vi "Write to Cell - Variant.vi"(8 "Column":i32=-1, 9 "Row":i32=-1, 10 "Value":variant, 11 "Excel Sheet in":refnum<class "Excel Sheet.lvclass">) -> (3 "Excel Sheet out":refnum<class "Excel Sheet.lvclass">)   [LabVIEW 2016, in "Excel Sheet.lvclass"]
uses:
  Excel Sheet.lvclass
  Excel Sheet.lvclass/Excel Sheet.ctl
panel:
  out "error out":errorcluster
  in  "error in (no error)":errorcluster
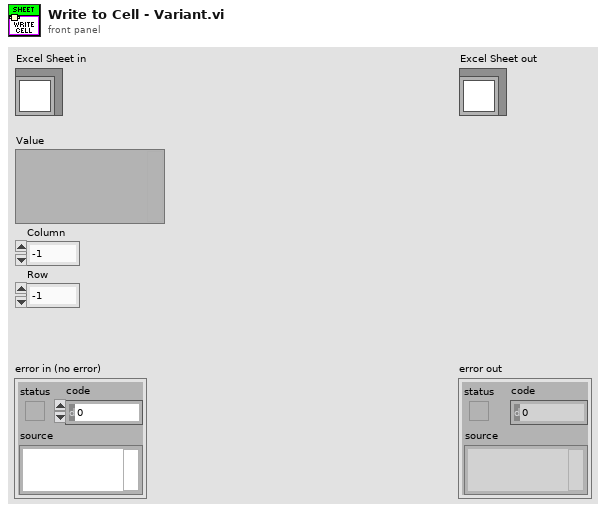
[diagram p1: front panel]
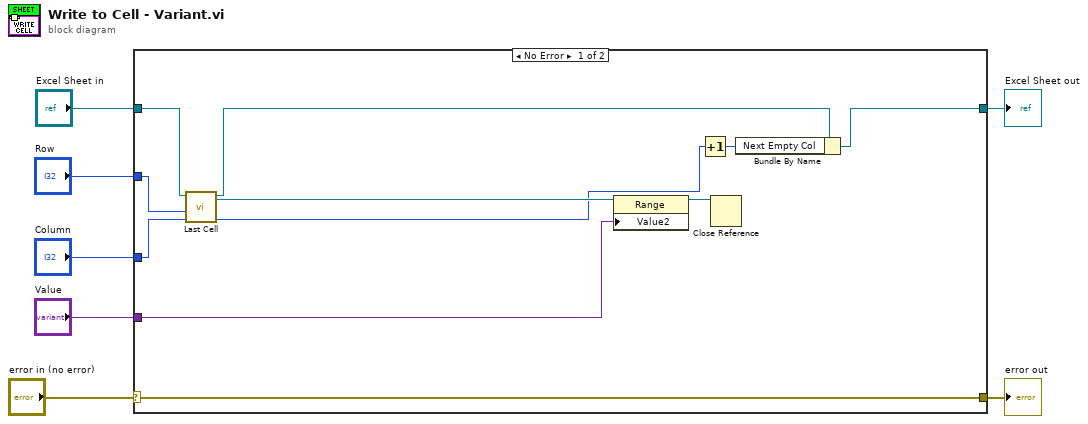
[diagram p0: block diagram]
diagram:
  n1 = case shown="No Error" "error in (no error)" {
    selector: "error in (no error)" -> [w18 w20]
    tunnel: [w18 w20] -> w6
    tunnel: [w16 w19] -> w4
    tunnel: "Excel Sheet in" -> [w13 w19]
    tunnel: "Column" -> [w10 _]
    tunnel: "Row" -> [w11 _]
    tunnel: "Value" -> [w17 _]
    frame No Error {
      n2 = call "Last Cell.vi"("Column"=w10, "Row"=w11, "Excel Sheet in"=w13) -> ("Column out"=w8:i32, "Cell"=w9:refnum<k7>, "Excel Sheet out"=w12:refnum<class "Excel Sheet.lvclass">)  [unwired: 5 in, 1 out]
      n3 = property class="Range"(reference=w9, "Value2"=w17) -> (reference out=w14:refnum<k7>)  [unwired: 1 in, 1 out]
      n4 = Increment(x=w8) -> (x+1=w15:i32)
      n5 = Close Reference(reference=w14) -> ()  [unwired: 1 in, 1 out]
      n6 = Bundle By Name(cluster=w12, "Next Empty Col"=w15) -> (w16:refnum<class "Excel Sheet.lvclass">)
    }
    frame Error {
    }
  }
  "error out" <- w6
  "Excel Sheet out" <- w4
